vi "UpdateElement(Single).vi"(7 "Qualified Name":string, 8 "error in (no error)":errorcluster, 9 "Value":string, 10 "Key":string, 11 "ConfigManager.Text.INI in":refnum<class "ConfigManager.Text.INI.lvclass">) -> (0 "error out":errorcluster, 3 "ConfigManager.Text.INI out":refnum<class "ConfigManager.Text.INI.lvclass">)   [LabVIEW 2013, in "CfgManager.Text.lvlib" / "ConfigManager.Text.INI.lvclass"]
uses:
  ConfigManager.Text.INI.lvclass
  Manager.Text/ConfigManager.Text.lvclass
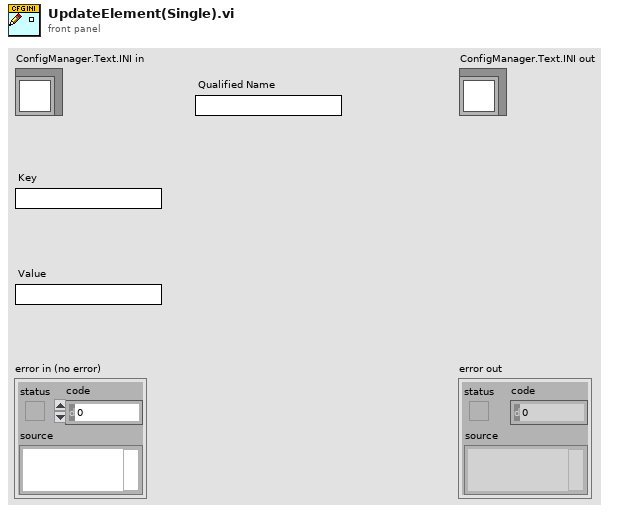
[diagram p1: front panel]
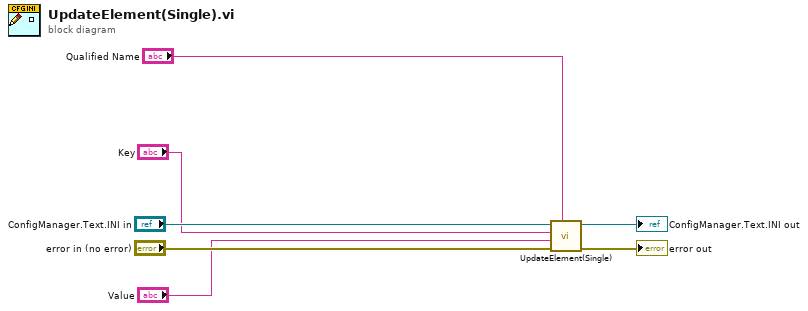
[diagram p0: block diagram]
diagram:
  n1 = call-parent "UpdateElement(Single).vi"("Qualified Name"="Qualified Name", "error in (no error)"="error in (no error)", "Value"="Value", "Key"="Key", "ConfigManager.Text in"="ConfigManager.Text.INI in") -> ("error out"=→"error out":errorcluster, "ConfigManager.Text out"=→"ConfigManager.Text.INI out":refnum<class "ConfigManager.Text.INI.lvclass">)  [unwired: 5 in]
